vi "Get ROI Col-Row.vi"(11 "Base Graph in":refnum<class "Base Graph.lvclass">) -> (2 "ROI Col-Row":T1, 3 "Base Graph out":refnum<class "Base Graph.lvclass">)   [LabVIEW 2025, in "Base Graph.lvclass"]
uses:
  Base Graph.lvclass
  Base Graph.lvclass/Base Graph.ctl
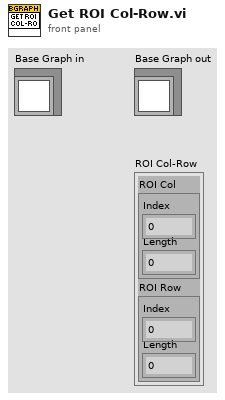
[diagram p1: front panel]
types:
  T1 = cluster{"ROI Col":cluster{"Index":u32, "Length":u32}, "ROI Row":cluster{"Index":u32, "Length":u32}}
  T2 = cluster{"ROI Cols":cluster{"Index":u32, "Length":u32}, "ROI Rows":cluster{"Index":u32, "Length":u32}}
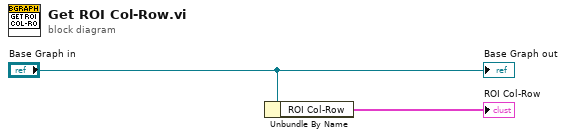
[diagram p0: block diagram]
diagram:
  n1 = Unbundle By Name("Base Graph in") -> ("ROI Col-Row"=→"ROI Col-Row":T2)
  "Base Graph out" <- "Base Graph in"
